vi "open_file_for_adam.vi"   [LabVIEW 2014]
types:
  T1 = enum16{"open", "replace", "create", "open or create", "replace or create", "replace or create with confirmation"}
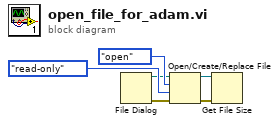
[diagram p0: block diagram]
diagram:
  n1 = File Dialog() -> (0:w3:errorcluster, 3:w1:path)  [unwired: 7 in, 2 out]
  n2 = Open/Create/Replace File(file path (use dialog)=w1, error in=w3, operation (0:open)=T1."open", access (0:read/write)=enum16{"read/write", "read-only", "write-only"}."read-only") -> (refnum out=w6:refnum<file>, error out=w2:errorcluster)  [unwired: 2 in, 1 out]
  n3 = Get File Size(file=w6, error in=w2) -> ()  [unwired: 3 out]
